vi "Configure Math.vi"   [LabVIEW 2010, in "Tektronix DPO MSO 2000 4000 Series.lvlib"]
doc: "The polymorphic VI configures math channel with different math operations.\nThe <B>tkdpo4k Configure Math (Dual)</B> VI configures a math channel for standard waveform math operations.\nThe <B>tkdpo4k Configure Math (FFT)</B> VI configures a math channel to calculate an FFT.\nThe <B>tkdpo4k Configure Math (Advanced)</B> VI configures a math channel using a mathematical expression.\nThe <B>tkdpo4k Configure Math (Spectrum)</B> VI configures a math channel\nto perform math operations on RF channels."
uses:
  <instrlib>/Tektronix DPO MSO 2000 4000 Series/Tektronix DPO MSO 2000 4000 Series.lvlib
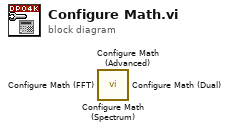
[diagram p0: block diagram]
diagram:
  n1 = call <instrlib>:"Configure Math (Spectrum).vi"() -> ()  [unwired: 10 in, 2 out]
  n2 = call <instrlib>:"Configure Math (Advanced).vi"() -> ()  [unwired: 10 in, 2 out]
  n3 = call <instrlib>:"Configure Math (FFT).vi"() -> ()  [unwired: 10 in, 2 out]
  n4 = call <instrlib>:"Configure Math (Dual).vi"() -> ()  [unwired: 10 in, 2 out]
